vi "create new assembly.vi"(8 "error in (no error)":errorcluster, 11 "EthernetIP configuration in":refnum<class "EthernetIP configuration.lvclass">) -> (0 "error out":errorcluster, 2 "assembly definition out":T1, 3 "EthernetIP configuration out":refnum<class "EthernetIP configuration.lvclass">)   [LabVIEW 2013, in "EthernetIP editor node.lvclass"]
uses:
  EthernetIP editor node.lvclass
  <vilib>/NI/TBM Modules/Ethernet IP/configuration/assembly definition.ctl
  <vilib>/NI/TBM Modules/Ethernet IP/configuration/assembly type.ctl
  <vilib>/NI/Tag Bus/tag/Data Type.ctl
  <vilib>/NI/TBM Modules/Ethernet IP/configuration/EthernetIP configuration.lvclass
  <vilib>/NI/TBM Modules/Ethernet IP/configuration/EthernetIP configuration.lvclass/EthernetIP configuration.ctl
  <vilib>/NI/TBM Modules/Ethernet IP/configuration/Read assemblies.vi
  <vilib>/NI/Tag Bus/tag/tag descriptor.lvclass
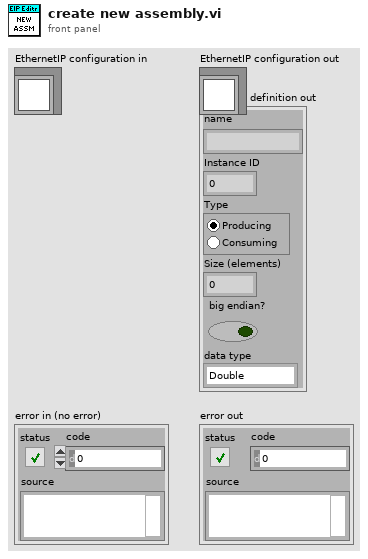
[diagram p1: front panel]
types:
  T1 = typedef "EthernetIP configuration.lvclass/assembly definition.ctl" = cluster{"name":string, "Instance ID":u32, "Type":T2, "Size (elements)":u32, "big endian?":bool, "data type":T3}
  T2 = typedef "EthernetIP configuration.lvclass/assembly type.ctl" = enum32{"Producing", "Consuming"}
  T3 = typedef "tag bus.lvlib/tag descriptor.lvclass/Data Type.ctl" = enum16{"Double", "Single", "I64", "I32", "I16", "I8", "U64", "U32", "U16", "U8", "Boolean", "String", "Array of Double", "Array of Single", "Array of I64", "Array of I32", "Array of I16", "Array of I8", "Array of U64", "Array of U32", "Array of U16", "Array of U8", "Array of Boolean", "Array of String"}
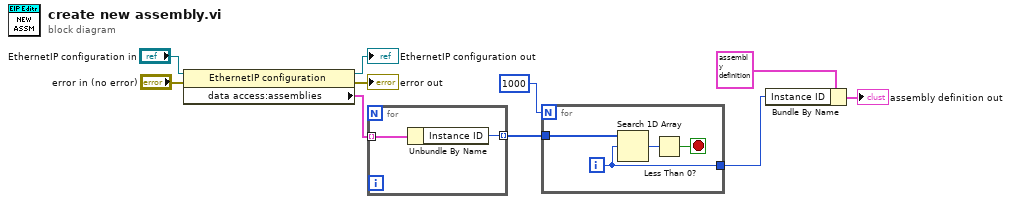
[diagram p0: block diagram]
diagram:
  n1 = property class="EthernetIP configuration"(reference="EthernetIP configuration in", error in="error in (no error)") -> (reference out=→"EthernetIP configuration out":refnum<class "EthernetIP configuration.lvclass">, error out=→"error out":errorcluster, "data access:assemblies"=w6:T1[])
  n2 = for {
    tunnel: w6 -> [w12] mode=indexing
    tunnel: [w11] -> w7 mode=indexing
    n3 = Unbundle By Name(w12) -> ("Instance ID"=w11:u32)
  }
  n4 = for {
    N: 1000 -> [_]
    tunnel: w7 -> [w16]
    tunnel: [w13] -> w10
    i -> [w13]
    stop <- w15 stop-if-true
    n5 = Search 1D Array(1D array=w16, element=w13) -> (index of element=w14:i32)  [unwired: 1 in]
    n6 = Less Than 0?(x=w14) -> (x < 0?=w15:bool)
  }
  n7 = Bundle By Name(cluster=T1 {"name"="", "Instance ID"=100, "Type"=enum."Producing", "Size (elements)"=32, "big endian?"=FALSE, "data type"=enum."Double"} ("assembly definition in"), "Instance ID"=w10) -> (→"assembly definition out":T1)
